vi "wavepond sequence.vi"(8 "Error In":errorcluster, 10 "Number of updates":i32) -> (0 "Error Out":errorcluster)   [LabVIEW 2014]
uses:
  Classes/D to A/Wavepond/Wavepond.lvclass
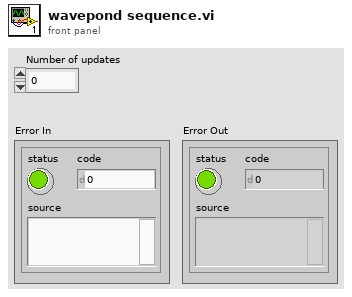
[diagram p1: front panel]
types:
  T1 = enum16{"Initialize", "SetFrequency", "SetAtten", "WriteData", "EnableSweep", "SetLoopCnt", "SetClkDiv", "SelExtTrig", "SoftTrig", "En_SqWave"}
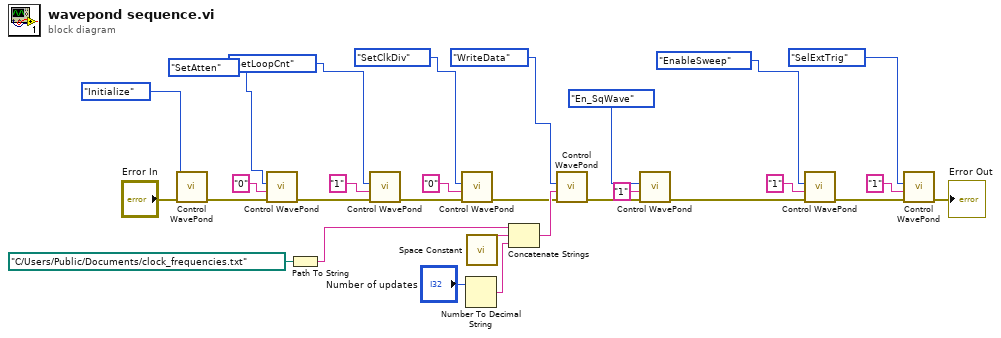
[diagram p0: block diagram]
diagram:
  n1 = call "Control WavePond.vi"("Error In"="Error In", "Command"=T1."Initialize") -> ("Error Out"=w28:errorcluster)  [unwired: 7 in, 2 out]
  n2 = call "Control WavePond.vi"("Error In"=w28, "Parameter"="0", "Command"=T1."SetAtten") -> ("Error Out"=w26:errorcluster)  [unwired: 6 in, 2 out]
  n3 = Path To String(path=path "C:/Users/Public/Documents/clock_frequencies.txt") -> (string=w16:string)
  n4 = call "Control WavePond.vi"("Error In"=w26, "Parameter"="1", "Command"=T1."SetLoopCnt") -> ("Error Out"=w24:errorcluster)  [unwired: 6 in, 2 out]
  n5 = call "Control WavePond.vi"("Error In"=w24, "Parameter"="0", "Command"=T1."SetClkDiv") -> ("Error Out"=w13:errorcluster)  [unwired: 6 in, 2 out]
  n6 = Number To Decimal String(number="Number of updates") -> (decimal integer string=w18:string)  [unwired: 1 in]
  n7 = call <vilib>:"Space Constant.vi"() -> ("String"=w17:string)
  n8 = Concatenate Strings(w16, w17, w18) -> (w23:string)
  n9 = call "Control WavePond.vi"("Error In"=w13, "Parameter"=w23, "Command"=T1."WriteData") -> ("Error Out"=w4:errorcluster)  [unwired: 6 in, 2 out]
  n10 = call "Control WavePond.vi"("Error In"=w4, "Parameter"="1", "Command"=T1."En_SqWave") -> ("Error Out"=w3:errorcluster)  [unwired: 6 in, 2 out]
  n11 = call "Control WavePond.vi"("Error In"=w3, "Parameter"="1", "Command"=T1."EnableSweep") -> ("Error Out"=w14:errorcluster)  [unwired: 6 in, 2 out]
  n12 = call "Control WavePond.vi"("Error In"=w14, "Parameter"="1", "Command"=T1."SelExtTrig") -> ("Error Out"=→"Error Out":errorcluster)  [unwired: 6 in, 2 out]
